vi "Convert Map To Array.vi"   [LabVIEW 2020]
doc: "Places the code that you can use to convert a map to an array."
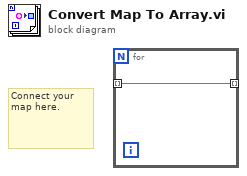
[diagram p0: block diagram]
diagram:
  # "Connect your map here."
  n1 = for {
    tunnel: [w1] -> _ mode=indexing
    tunnel: _ -> [w1] mode=indexing
  }
